vi "Write Button Properties.vi"(8 "error in (no error)":errorcluster, 10 "Button":T1, 11 "RunTimeButton in":refnum<class "RunTimeButton.lvclass">) -> (0 "error out":errorcluster, 3 "RunTimeButton out":refnum<class "RunTimeButton.lvclass">)   [LabVIEW 2019, in "RunTimeButton.lvclass"]
uses:
  RunTimeButton.lvclass
  XML Controls/ButtonLists Properties.ctl
  XML Controls/Path Cluster.ctl
  XML Controls/Button Type.ctl
  XML Controls/Dependency Properties.ctl
  RunTimeButton.lvclass/RunTimeButton.ctl
  VeriStand Custom Device XML Parser.lvlib
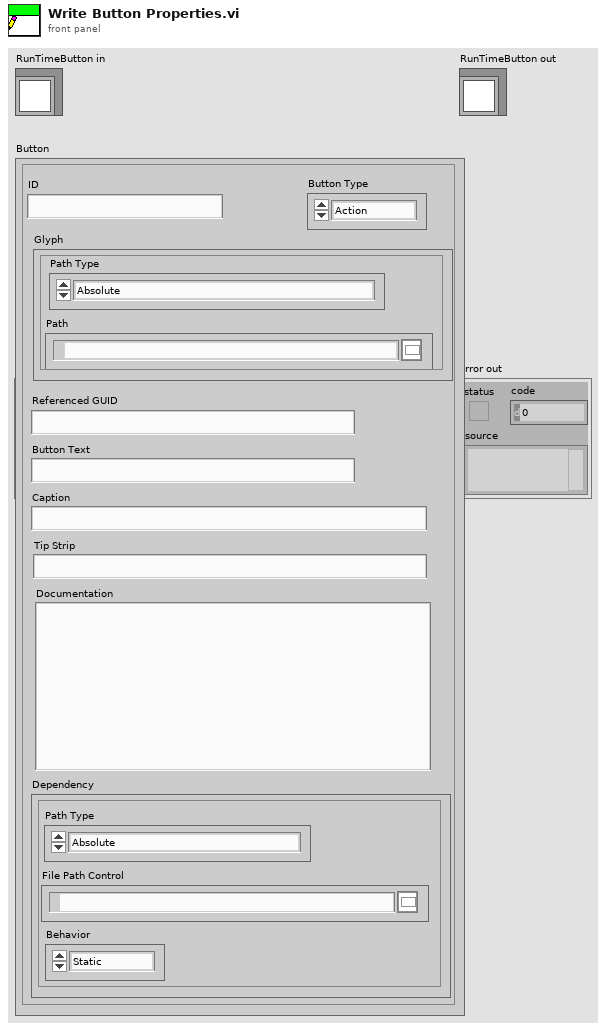
[diagram p1: front panel]
types:
  T1 = typedef "VeriStand Custom Device XML Parser.lvlib/ButtonLists Properties.ctl" = cluster{"ID":string, "Glyph":T2, "Button Type":T3, "Referenced GUID":string, "Button Text":string, "Caption":string, "Tip Strip":string, "Documentation":string, "Dependency":T4}
  T2 = typedef "VeriStand Custom Device XML Parser.lvlib/Path Cluster.ctl" = cluster{"Path":path, "Path Type":enum16{"Absolute", "To Base", "To Common Doc Dir", "To Application Data Dir"}}
  T3 = typedef "VeriStand Custom Device XML Parser.lvlib/Button Type.ctl" = enum16{"Action", "Dialog", "Page", "Notification", "Separator"}
  T4 = typedef "VeriStand Custom Device XML Parser.lvlib/Dependency Properties.ctl" = cluster{"File Path Control":path, "Path Type":enum16{"Absolute", "To Base", "To Common Doc Dir", "To Application Data Dir"}, "Behavior":enum16{"Static", "Dynamic"}}
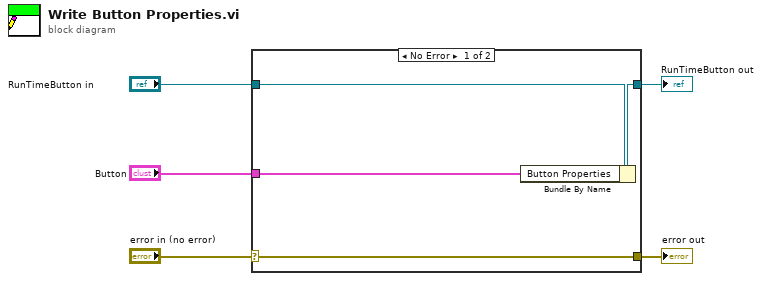
[diagram p0: block diagram]
diagram:
  n1 = case shown="No Error" "error in (no error)" {
    selector: "error in (no error)" -> [w9 w10]
    tunnel: [w9 w10] -> w4
    tunnel: [w7 w11] -> w2
    tunnel: "RunTimeButton in" -> [w8 w11]
    tunnel: "Button" -> [w6 _]
    frame No Error {
      n2 = Bundle By Name(cluster=w8, "Button Properties"=w6) -> (w7:refnum<class "RunTimeButton.lvclass">)
    }
    frame Error {
    }
  }
  "error out" <- w4
  "RunTimeButton out" <- w2
